vi "1D Array (Sine+Normal).vi"(0 "Amplitude":dbl=1.0, 1 "Frequency":dbl=1.0, 2 "Sample Rate":dbl=10.0, 3 "interpolation_degree":i32, 4 "Signal Length":dbl=10.0, 5 "Noise Amplitude":dbl=0.1, 6 "Phase (degrees)":dbl=90.0, 7 "fixed seed":bool=TRUE, 9 "seed":i32=172) -> (15 "y(t)":dbl[](array[numeric])=[0.9835342378358874, 0.8533662731765123, 0.1935938445391167, -0.2180566832246157, -0.8820527242230749, -0.8532198097671811, -0.9096526006201997, -0.4441140263754137, 0.5007139304552086, 0.8694858451498179, 0.8944953349515332, 0.7751438451748646, 0.3178316536450238, -0.2166598580218596, -0.7846019921742773, -1.0290774357839088, -0.8123101389888427, -0.056100517834243635, 0.3730775035346127, 0.8025254867763597, 0.9990546652886879, 0.8998025404550115, 0.3537461122093949, -0.177301546960321, -0.6986482436835849, -1.0608986815819563, -0.9691831386987784, -0.4332175862058382, 0.29384196147460295, 0.8823384099061323, 0.8814913743417987, 0.7554750631366305, 0.39244797661994685, -0.0649333698000586, -0.6908841065826775, -1.1005762654551396, -0.7308778081813541, -0.3575291596832779, 0.268597958855942, 0.5963135557055195, 1.0131561594257588, 0.9099367107833473, 0.12684364291193406, -0.23612254823391993, -0.7723189603836355, -1.0873776907507746, -0.9311967611668752, -0.27332076015807044, 0.3335001132129122, 0.670794311347244, 1.0747282226122503, 0.6921202875821097, 0.14231261059114558, -0.1782959058841038, -0.8729711440161438, -0.9343658008323608, -0.7034755428980883, -0.4069785218584952, 0.46804498281147555, 0.7571563026466923, 0.7443028541822899, 0.6422047007451028, 0.1698031570325397, -0.3933458794604654, -0.6707839071317667, -1.05747180995087, -0.8823220261319941, -0.375371330015255, 0.3788701911413331, 0.6750111028323957, 1.17948877103449, 0.8410220526292967, 0.3365656183934219, -0.4179030097685975, -0.7805169545958929, -1.0062470833712878, -0.8402069550792994, -0.21705186084860412, 0.22549861423224643, 0.9292527670427374, 0.9915710152050596, 0.7006928728611147, 0.4088981275835714, -0.35087665529163936, -0.8182187891082517, -0.8838013880161452, -0.8336076539633117, -0.17937828753371854, 0.37204887254038943, 0.7826552495642436, 1.060796712544878, 0.8424956023462578, 0.3840654387920989, -0.32477714642960404, -0.8768761651241542, -1.0112147606820523, -0.6188831855335302, -0.37010741564874905, 0.248296706105914, 0.7478683484637981, 0.9474066454065756] format="%_6g", 18 "t":dbl[](array[numeric])=[0.0, 1.0, 2.0, 3.0, 4.0, 5.0, 6.0, 7.0, 8.0, 9.0, 10.0, 11.0, 12.0, 13.0, 14.0, 15.0, 16.0, 17.0, 18.0, 19.0, 20.0, 21.0, 22.0, 23.0, 24.0, 25.0, 26.0, 27.0, 28.0, 29.0, 30.0, 31.0, 32.0, 33.0, 34.0, 35.0, 36.0, 37.0, 38.0, 39.0, 40.0, 41.0, 42.0, 43.0, 44.0, 45.0, 46.0, 47.0, 48.0, 49.0, 50.0, 51.0, 52.0, 53.0, 54.0, 55.0, 56.0, 57.0, 58.0, 59.0, 60.0, 61.0, 62.0, 63.0, 64.0, 65.0, 66.0, 67.0, 68.0, 69.0, 70.0, 71.0, 72.0, 73.0, 74.0, 75.0, 76.0, 77.0, 78.0, 79.0, 80.0, 81.0, 82.0, 83.0, 84.0, 85.0, 86.0, 87.0, 88.0, 89.0, 90.0, 91.0, 92.0, 93.0, 94.0, 95.0, 96.0, 97.0, 98.0, 99.0, 100.0] format="%_6g", 19 "points_per_cycle = (sample_rate) * 2^(interpolation_degree) + (Frequency/Signal_Length)":dbl=10.1)   [LabVIEW 2014]
uses:
  <vilib>/gmath/NI_Gmath.lvlib
panel:
  out "Raw":T1(graph)={"Scaled 1D Array"=[0.0, 1.0, 2.0, 3.0, 4.0, 5.0, 6.0, 7.0, 8.0, 9.0, 10.0, 11.0, 12.0, 13.0, 14.0, 15.0, 16.0, 17.0, 18.0, 19.0, 20.0, 21.0, 22.0, 23.0, 24.0, 25.0, 26.0, 27.0, 28.0, 29.0, 30.0, 31.0, 32.0, 33.0, 34.0, 35.0, 36.0, 37.0, 38.0, 39.0, 40.0, 41.0, 42.0, 43.0, 44.0, 45.0, 46.0, 47.0, 48.0, 49.0, 50.0, 51.0, 52.0, 53.0, 54.0, 55.0, 56.0, 57.0, 58.0, 59.0, 60.0, 61.0, 62.0, 63.0, 64.0, 65.0, 66.0, 67.0, 68.0, 69.0, 70.0, 71.0, 72.0, 73.0, 74.0, 75.0, 76.0, 77.0, 78.0, 79.0, 80.0, 81.0, 82.0, 83.0, 84.0, 85.0, 86.0, 87.0, 88.0, 89.0, 90.0, 91.0, 92.0, 93.0, 94.0, 95.0, 96.0, 97.0, 98.0, 99.0, 100.0], "Scaled 1D Array"=[0.9835342378358874, 0.8533662731765123, 0.1935938445391167, -0.2180566832246157, -0.882052724223075, -0.8532198097671811, -0.9096526006201997, -0.4441140263754137, 0.5007139304552086, 0.8694858451498179, 0.8944953349515332, 0.7751438451748646, 0.3178316536450238, -0.2166598580218596, -0.7846019921742773, -1.0290774357839088, -0.8123101389888427, -0.056100517834243635, 0.3730775035346127, 0.8025254867763597, 0.9990546652886878, 0.8998025404550115, 0.3537461122093949, -0.177301546960321, -0.6986482436835849, -1.0608986815819563, -0.9691831386987784, -0.4332175862058382, 0.29384196147460295, 0.8823384099061323, 0.8814913743417987, 0.7554750631366305, 0.39244797661994685, -0.0649333698000586, -0.6908841065826775, -1.1005762654551396, -0.7308778081813541, -0.3575291596832779, 0.268597958855942, 0.5963135557055195, 1.0131561594257588, 0.9099367107833471, 0.12684364291193406, -0.23612254823391993, -0.7723189603836355, -1.0873776907507746, -0.9311967611668751, -0.27332076015807044, 0.3335001132129122, 0.670794311347244, 1.0747282226122503, 0.6921202875821097, 0.14231261059114558, -0.1782959058841038, -0.8729711440161438, -0.9343658008323608, -0.7034755428980883, -0.40697852185849526, 0.46804498281147555, 0.7571563026466923, 0.7443028541822899, 0.6422047007451028, 0.1698031570325397, -0.3933458794604654, -0.6707839071317667, -1.05747180995087, -0.8823220261319941, -0.375371330015255, 0.37887019114133313, 0.6750111028323957, 1.17948877103449, 0.8410220526292967, 0.3365656183934219, -0.4179030097685975, -0.7805169545958929, -1.006247083371288, -0.8402069550792994, -0.21705186084860412, 0.22549861423224643, 0.9292527670427374, 0.9915710152050596, 0.7006928728611147, 0.40889812758357136, -0.35087665529163936, -0.8182187891082517, -0.8838013880161452, -0.8336076539633116, -0.17937828753371854, 0.37204887254038943, 0.7826552495642436, 1.060796712544878, 0.8424956023462578, 0.3840654387920989, -0.32477714642960404, -0.8768761651241542, -1.0112147606820523, -0.6188831855335302, -0.37010741564874905, 0.248296706105914, 0.7478683484637981, 0.9474066454065756]}
  out "Interpolated":cluster{"xi used":dbl[], "yi":dbl[]}(graph)={"xi used"=[0.0, 1.0, 2.0, 3.0, 4.0, 5.0, 6.0, 7.0, 8.0, 9.0, 10.0, 11.0, 12.0, 13.0, 14.0, 15.0, 16.0, 17.0, 18.0, 19.0, 20.0, 21.0, 22.0, 23.0, 24.0, 25.0, 26.0, 27.0, 28.0, 29.0, 30.0, 31.0, 32.0, 33.0, 34.0, 35.0, 36.0, 37.0, 38.0, 39.0, 40.0, 41.0, 42.0, 43.0, 44.0, 45.0, 46.0, 47.0, 48.0, 49.0, 50.0, 51.0, 52.0, 53.0, 54.0, 55.0, 56.0, 57.0, 58.0, 59.0, 60.0, 61.0, 62.0, 63.0, 64.0, 65.0, 66.0, 67.0, 68.0, 69.0, 70.0, 71.0, 72.0, 73.0, 74.0, 75.0, 76.0, 77.0, 78.0, 79.0, 80.0, 81.0, 82.0, 83.0, 84.0, 85.0, 86.0, 87.0, 88.0, 89.0, 90.0, 91.0, 92.0, 93.0, 94.0, 95.0, 96.0, 97.0, 98.0, 99.0, 100.0], "yi"=[0.9835342378358874, 0.8533662731765123, 0.1935938445391167, -0.2180566832246157, -0.8820527242230749, -0.8532198097671811, -0.9096526006201997, -0.4441140263754137, 0.5007139304552086, 0.8694858451498179, 0.8944953349515332, 0.7751438451748646, 0.3178316536450238, -0.2166598580218596, -0.7846019921742773, -1.0290774357839088, -0.8123101389888427, -0.056100517834243635, 0.3730775035346127, 0.8025254867763597, 0.9990546652886879, 0.8998025404550115, 0.3537461122093949, -0.177301546960321, -0.6986482436835849, -1.0608986815819563, -0.9691831386987784, -0.4332175862058382, 0.29384196147460295, 0.8823384099061323, 0.8814913743417987, 0.7554750631366305, 0.39244797661994685, -0.0649333698000586, -0.6908841065826775, -1.1005762654551396, -0.7308778081813541, -0.3575291596832779, 0.268597958855942, 0.5963135557055195, 1.0131561594257588, 0.9099367107833473, 0.12684364291193406, -0.23612254823391993, -0.7723189603836355, -1.0873776907507746, -0.9311967611668752, -0.27332076015807044, 0.3335001132129122, 0.670794311347244, 1.0747282226122503, 0.6921202875821097, 0.14231261059114558, -0.1782959058841038, -0.8729711440161438, -0.9343658008323608, -0.7034755428980883, -0.4069785218584952, 0.46804498281147555, 0.7571563026466923, 0.7443028541822899, 0.6422047007451028, 0.1698031570325397, -0.3933458794604654, -0.6707839071317667, -1.05747180995087, -0.8823220261319941, -0.375371330015255, 0.3788701911413331, 0.6750111028323957, 1.17948877103449, 0.8410220526292967, 0.3365656183934219, -0.4179030097685975, -0.7805169545958929, -1.0062470833712878, -0.8402069550792994, -0.21705186084860412, 0.22549861423224643, 0.9292527670427374, 0.9915710152050596, 0.7006928728611147, 0.4088981275835714, -0.35087665529163936, -0.8182187891082517, -0.8838013880161452, -0.8336076539633117, -0.17937828753371854, 0.37204887254038943, 0.7826552495642436, 1.060796712544878, 0.8424956023462578, 0.3840654387920989, -0.32477714642960404, -0.8768761651241542, -1.0112147606820523, -0.6188831855335302, -0.37010741564874905, 0.248296706105914, 0.7478683484637981, 0.9474066454065756]}
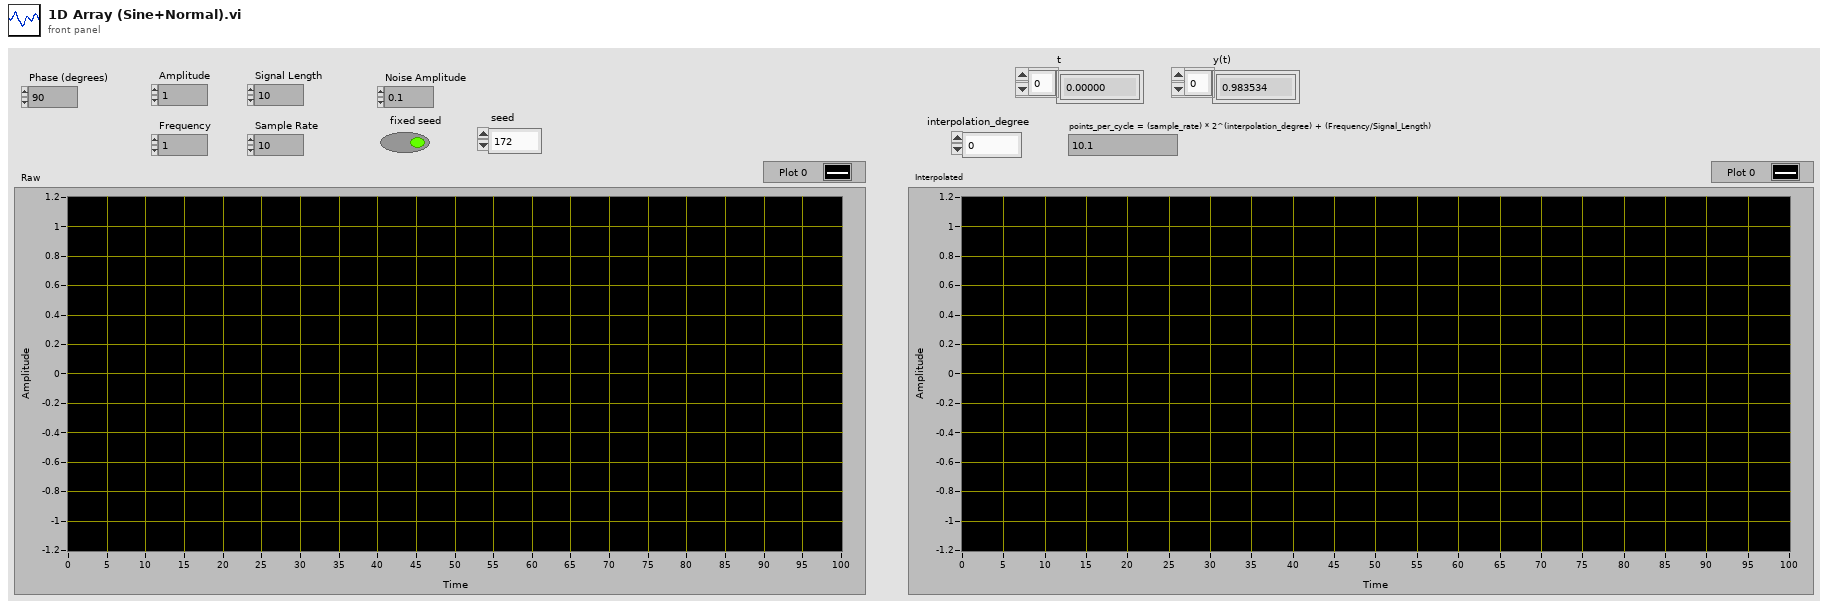
[diagram p1: front panel]
types:
  T1 = cluster{"Scaled 1D Array":dbl[], "Scaled 1D Array":dbl[]}
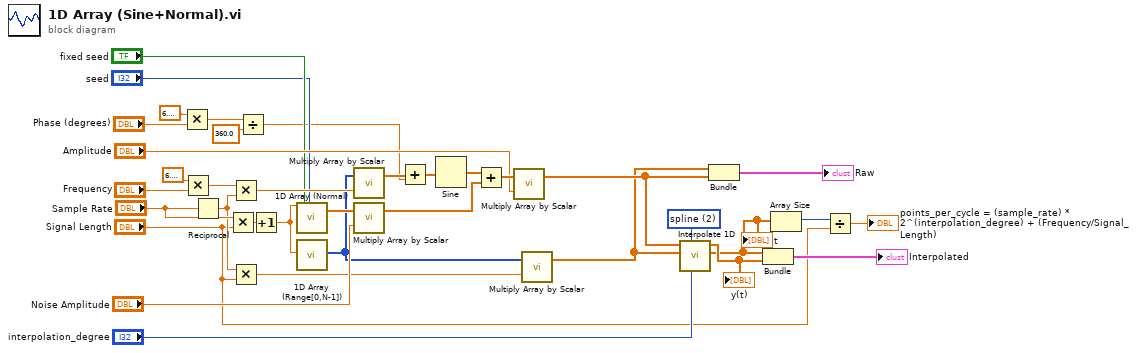
[diagram p0: block diagram]
diagram:
  w36 = 2 items=["nearest", "linear", "spline", "cubic Hermite", "Lagrange"] ("method")
  n1 = Multiply(x=6.283185307179586, y="Phase (degrees)") -> (x*y=w3:dbl)
  n2 = Multiply(x=6.283185307179586, y="Frequency") -> (x*y=w20:dbl)
  n3 = Reciprocal(x="Sample Rate") -> (1/x=w12:dbl)
  n4 = Multiply(x="Sample Rate", y="Signal Length") -> (x*y=w19:dbl)
  n5 = Multiply(x=w20, y=w12) -> (x*y=w31:dbl)
  n6 = Multiply(x=w12, y="Signal Length") -> (x*y=w11:dbl)
  n7 = Divide(x=w3, y=360.0) -> (x/y=w1:dbl)
  n8 = Increment(x=w19) -> (x+1=w16:dbl)
  n9 = call "1D Array (Normal).vi"("samples"=w16, "fixed seed"="fixed seed", "seed"="seed") -> ("normal random data"=w25:dbl[])  [unwired: 16 in]
  n10 = call "1D Array (Range[0,N-1]).vi"("Range"=w16) -> ("Array"=w14:i32[])  [unwired: 18 in]
  n11 = call "Multiply Array by Scalar.vi"("1D Array"=w14, "Scaling Factor"=w31) -> ("Scaled 1D Array"=w7:dbl[])  [unwired: 17 in]
  n12 = call "Multiply Array by Scalar.vi"("1D Array"=w25, "Scaling Factor"="Noise Amplitude") -> ("Scaled 1D Array"=w26:dbl[])  [unwired: 17 in]
  n13 = Add(x=w7, y=w1) -> (x+y=w6:dbl[])
  n14 = Sine(x=w6) -> (sin(x)=w32:dbl[])
  n15 = Add(x=w32, y=w26) -> (x+y=w29:dbl[])
  n16 = call "Multiply Array by Scalar.vi"("1D Array"=w29, "Scaling Factor"="Amplitude") -> ("Scaled 1D Array"=w27:dbl[])  [unwired: 17 in]
  n17 = call "Multiply Array by Scalar.vi"("1D Array"=w14, "Scaling Factor"=w11) -> ("Scaled 1D Array"=w13:dbl[])  [unwired: 17 in]
  n18 = call <vilib>:"Interpolate 1D.vi"("ntimes"="interpolation_degree", "method"=w36, "X"=w13, "Y"=w27) -> ("xi used"=w18:dbl[], "yi"=w35:dbl[])  [unwired: 5 in, 1 out]
  "t" <- w18
  "y(t)" <- w35
  n19 = Bundle("Scaled 1D Array"=w13, "Scaled 1D Array"=w27) -> (→"Raw":T1)  [unwired: 1 in]
  n20 = Bundle("xi used"=w18, "yi"=w35) -> (→"Interpolated":cluster{"xi used":dbl[], "yi":dbl[]})  [unwired: 1 in]
  n21 = Array Size(array=w18) -> (size(s)=w17:i32)
  n22 = Divide(x=w17, y="Signal Length") -> (x/y=→"points_per_cycle = (sample_rate) * 2^(interpolation_degree) + (Frequency/Signal_Length)":dbl)
